vi "Overtones.vi"() -> ()   [LabVIEW 2023]
uses:
  <vilib>/sound2/lvsound2.llb/Sound Data Format.ctl
  <vilib>/sound2/lvsound2.llb/Sampling Mode.ctl
  <vilib>/sound2/lvsound2.llb/Sound Input Read (DBL).vi
  <vilib>/Analysis/NI_AALPro.lvlib
panel:
  in  "path":path
  out "Spectrum":waveform(dbl)(graph)
  out "Data":waveform(dbl)[](graph)
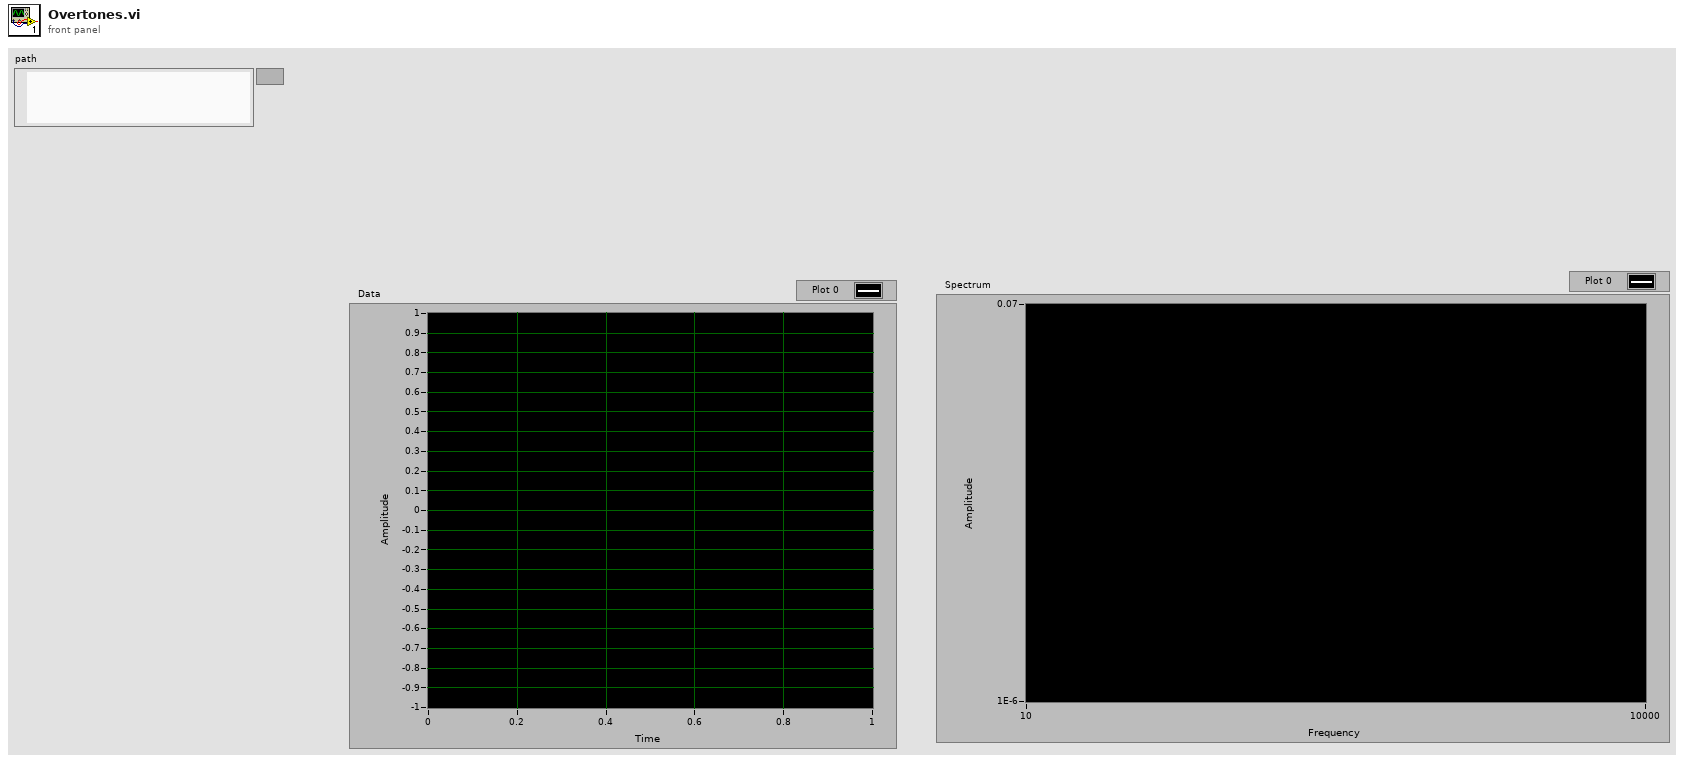
[diagram p1: front panel]
types:
  T1 = typedef "Sampling Mode.ctl" = i32
  T2 = typedef "Sound Data Format.ctl" = cluster{"sample rate (S/s)":dbl, "number of channels":i32, "bits per sample":i32}
  T3 = typedef "Sound Input Task ID.ctl" = u32
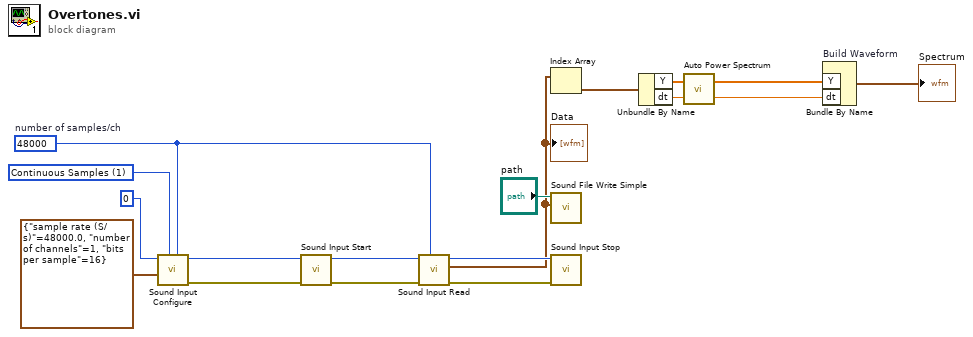
[diagram p0: block diagram]
diagram:
  w10 = 48000  # number of samples/ch
  w11 = T1 1 items=["Finite Samples", "Continuous Samples"] ("sample mode")
  n1 = call <vilib>:"Sound Input Configure.vi"("number of samples/ch"=w10, "sample mode"=w11, "sound format"=T2 {"sample rate (S/s)"=48000.0, "number of channels"=1, "bits per sample"=16}, "device ID"=u32 0) -> ("error out"=w16:errorcluster, "task ID"=w18:T3)  [unwired: 6 in]
  n2 = call <vilib>:"Sound Input Start.vi"("error in (no error)"=w16, "task ID"=w18) -> ("error out"=w14:errorcluster, "task ID out"=w15:T3)  [unwired: 8 in]
  n3 = call-poly <vilib>:"Sound Input Read.vi"("number of samples/ch"=w10, "error in (no error)"=w14, "task ID"=w15) -> ("error out"=w13:errorcluster, "data"=w1:waveform(dbl)[], "task ID out"=w9:T3)  [unwired: 6 in]
  "Data" <- w1
  n4 = Index Array "Index Array"(array=w1) -> (element=w8:waveform(dbl))  [unwired: 1 in]
  n5 = call <vilib>:"Sound File Write Simple.vi"("data"=w1, "path"="path") -> ()  [unwired: 8 in, 2 out]
  n6 = call <vilib>:"Sound Input Stop.vi"("error in (no error)"=w13, "task ID"=w9) -> ()  [unwired: 8 in, 2 out]
  n7 = Unbundle By Name(w8) -> ("Y"=w7:dbl[], "dt"=w6:dbl)
  n8 = call <vilib>:"Auto Power Spectrum.vi"("dt"=w6, "Signal (V)"=w7) -> ("df"=w5:dbl, "Power Spectrum (V^2 rms)"=w4:dbl[])
  n9 = Bundle By Name "Build Waveform"("Y"=w4, "dt"=w5) -> (→"Spectrum":waveform(dbl))  [unwired: 1 in]
